vi "do_waveform_full.vi"() -> ()   [LabVIEW 2020]
uses:
  <vilib>/Waveform/DWDTOps.llb/DWDT Analog to Digital.vi
panel:
  out "数字波形图":digitalwaveform(graph)={"t0"=timestamp(0 s since 1904-01-01), "dt"=1e-05, "Y"={"transitions"=[0, 1, 2, 3, 4, 5], "data"=[[0, 0, 0, 0], [0, 1, 0, 1], [1, 0, 1, 0], [0, 0, 0, 1], [1, 0, 0, 1], [0, 0, 0, 0]]}}
  in  "Value":u32[](array[numeric])=[0, 13, 2, 9, 0, 9] format="%04b"
  in  "DoCycle":u32=1
  out "error out":errorcluster caption="错误输出"
  in  "SamplePeriod(ns)":u32=10000
  in  "DevIndex":i32
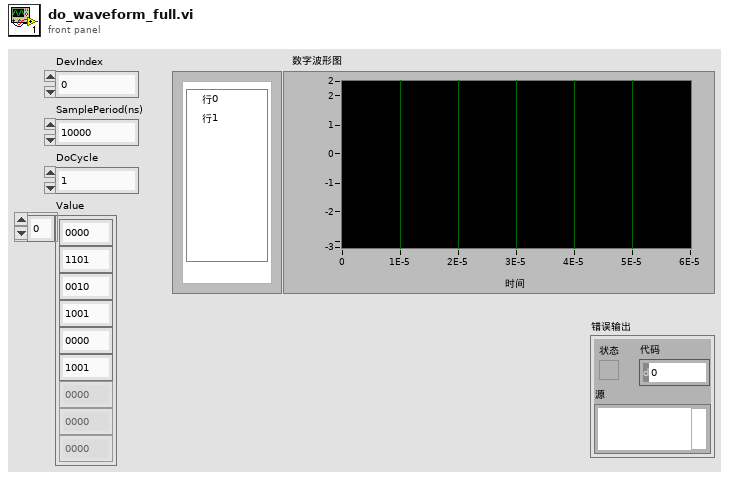
[diagram p1: front panel]
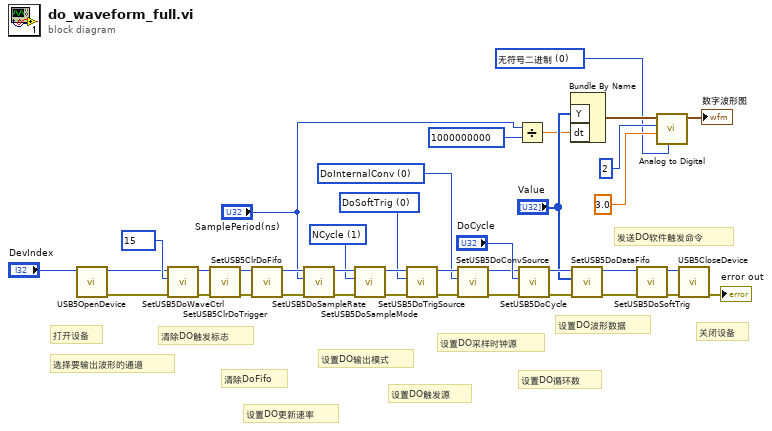
[diagram p0: block diagram]
diagram:
  w1 = u8 0 items=["DoInternalConv"=0, "ConvIn"=1, "AiConv"=2, "DiConv"=3, "Ao0Conv"=5, "Ao1Conv"=6, "Ao2Conv"=7, "Ao3Conv"=8] ("DoConvSource")
  w2 = u8 0 items=["DoSoftTrig"=0, "ExtTrigIn"=1, "Din0RisingEdge"=2, "Din1RisingEdge"=3, "Din2RisingEdge"=4, "Din3RisingEdge"=5, "WithAiTrig"=6, "WithDiTrig"=7, "WithAo0Trig"=9, "WithAo1Trig"=10, "WithAo2Trig"=11, "WithAo3Trig"=12, "GlobalSoftTrig"=255] ("DoTrigSource")
  w3 = u8 1 items=["PcBufferedInfinite", "NCycle"] ("DoSampleMode")
  w21 = u16 0 items=["无符号二进制", "二进制偏移量", "二进制补码"] ("data format (offset binary)")
  # "关闭设备"
  # "发送DO软件触发命令"
  # "设置DO波形数据"
  # "设置DO循环数"
  # "设置DO采样时钟源"
  # "设置DO触发源"
  # "设置DO输出模式"
  # "设置DO更新速率"
  # "清除DoFifo"
  # "清除DO触发标志"
  # "选择要输出波形的通道"
  # "打开设备"
  n1 = call "USB5OpenDevice.vi"("DevIndex"="DevIndex") -> ("error out"=w5:errorcluster, "DevIndex Out"=w6:i32)  [unwired: 9 in]
  n2 = call "SetUSB5DoWaveCtrl.vi"("错误输入（无错误）"=w5, "Chan"=u32 15, "DevIndex"=w6) -> ("错误输出"=w16:errorcluster, "DevIndex Out"=w17:i32)  [unwired: 7 in]
  n3 = call "SetUSB5ClrDoTrigger.vi"("错误输入（无错误）"=w16, "DevIndex"=w17) -> ("错误输出"=w35:errorcluster, "DevIndex Out"=w36:i32)  [unwired: 8 in]
  n4 = call "SetUSB5ClrDoFifo.vi"("错误输入（无错误）"=w35, "DevIndex"=w36) -> ("错误输出"=w33:errorcluster, "DevIndex Out"=w34:i32)  [unwired: 8 in]
  n5 = call "SetUSB5DoSampleRate.vi"("错误输入（无错误）"=w33, "SamplePeriod(ns)"="SamplePeriod(ns)", "DevIndex"=w34) -> ("错误输出"=w13:errorcluster, "DevIndex Out"=w14:i32)  [unwired: 7 in]
  n6 = call "SetUSB5DoSampleMode.vi"("错误输入（无错误）"=w13, "DoSampleMode"=w3, "DevIndex"=w14) -> ("错误输出"=w11:errorcluster, "DevIndex Out"=w12:i32)  [unwired: 7 in]
  n7 = call "SetUSB5DoTrigSource.vi"("错误输入（无错误）"=w11, "DoTrigSource"=w2, "DevIndex"=w12) -> ("错误输出"=w9:errorcluster, "DevIndex Out"=w10:i32)  [unwired: 7 in]
  n8 = call "SetUSB5DoConvSource.vi"("错误输入（无错误）"=w9, "DoConvSource"=w1, "DevIndex"=w10) -> ("错误输出"=w7:errorcluster, "DevIndex Out"=w8:i32)  [unwired: 7 in]
  n9 = Divide(x="SamplePeriod(ns)", y=u32 1000000000) -> (x/y=w18:dbl)
  n10 = call "SetUSB5DoCycle.vi"("错误输入（无错误）"=w7, "DoCycle"="DoCycle", "DevIndex"=w8) -> ("错误输出"=w30:errorcluster, "DevIndex Out"=w31:i32)  [unwired: 7 in]
  n11 = Bundle By Name ("创建波形")("Y"="Value", "dt"=w18) -> (w24:waveform(u32))  [unwired: 1 in]
  n12 = call "SetUSB5DoDataFifo.vi"("错误输入（无错误）"=w30, "Value"="Value", "DevIndex"=w31) -> ("错误输出"=w28:errorcluster, "DevIndex Out"=w29:i32)  [unwired: 7 in]
  n13 = call "SetUSB5DoSoftTrig.vi"("错误输入（无错误）"=w28, "DevIndex"=w29) -> ("错误输出"=w26:errorcluster, "DevIndex Out"=w27:i32)  [unwired: 8 in]
  n14 = call-poly <vilib>:"Analog to Digital.vi"("data format (offset binary)"=w21, "full-scale range (pk-pk)"=3.0, "resolution (16 bit)"=2, "analog waveform"=w24) -> ("digital waveform"=→"数字波形图":digitalwaveform)  [unwired: 4 in, 3 out]
  n15 = call "USB5CloseDevice.vi"("错误输入（无错误）"=w26, "DevIndex"=w27) -> ("error out"=→"error out":errorcluster)  [unwired: 8 in, 1 out]
